vi "PDash - Rename DQMH Module.vi"(9 "New Module Library":path, 10 "Module Info (old)":T1, 11 "Project":refnum<vi>) -> (0 "error out":errorcluster)   [LabVIEW 2019]
doc: "_____\nCreated using DQMH Event Scripter 7.1.0.1447."
uses:
  PantherDashboard Scripting Hooks/Panther Dasboard Scripting Hooks.lvlib
  <vilib>/Delacor/Delacor QMH/Libraries/_Scripting Support/Module Type--enum.ctl
  <vilib>/Delacor/Delacor QMH/Libraries/_Scripting Support/dqmh_lib_DQMH Scripting Support.lvlib
  <vilib>/Delacor/Delacor QMH/Libraries/_Scripting Support/Module Info--cluster.ctl
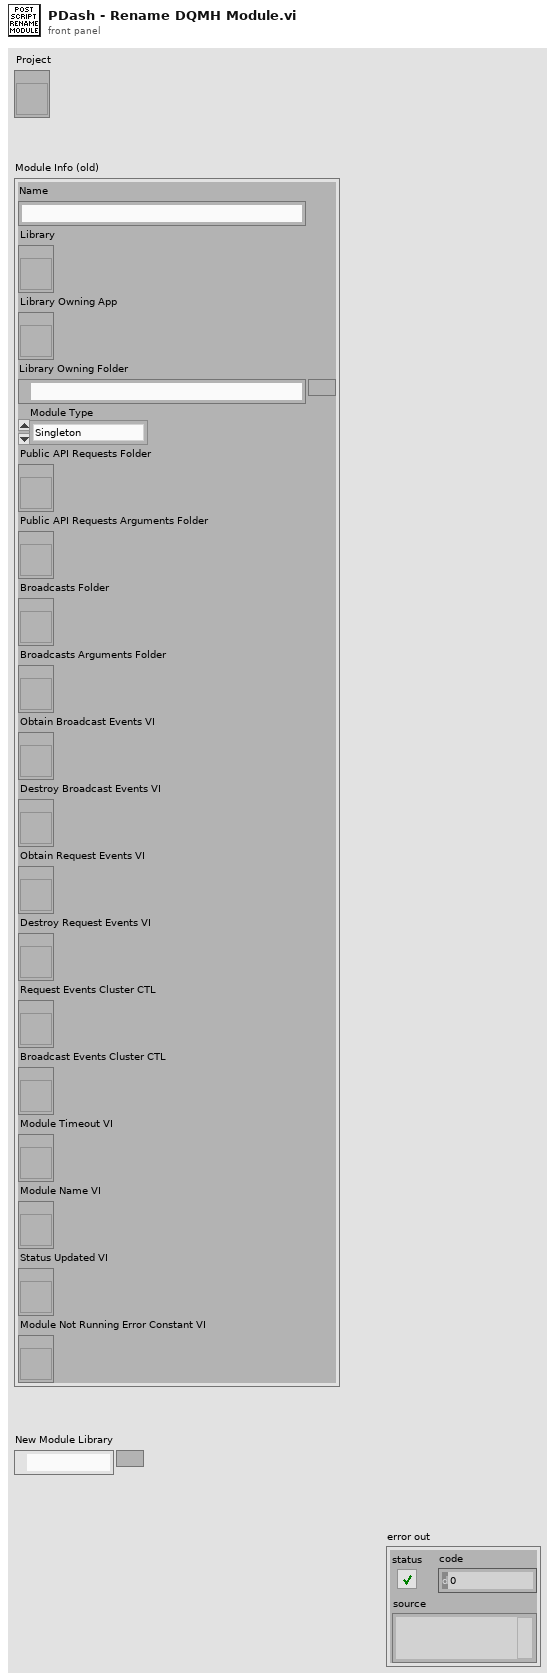
[diagram p1: front panel]
types:
  T1 = typedef "dqmh_lib_DQMH Scripting Support.lvlib/Module Info--cluster.ctl" = cluster{"Name":string, "Library":refnum<vi>, "Library Owning App":refnum<vi>, "Library Owning Folder":path, "Module Type":T2, "Public API Requests Folder":refnum<vi>, "Public API Requests Arguments Folder":refnum<vi>, "Broadcasts Folder":refnum<vi>, "Broadcasts Arguments Folder":refnum<vi>, "Obtain Broadcast Events VI":refnum<vi>, "Destroy Broadcast Events VI":refnum<vi>, "Obtain Request Events VI":refnum<vi>, "Destroy Request Events VI":refnum<vi>, "Request Events Cluster CTL":refnum<vi>, "Broadcast Events Cluster CTL":refnum<vi>, "Module Timeout VI":refnum<vi>, "Module Name VI":refnum<vi>, "Status Updated VI":refnum<vi>, "Module Not Running Error Constant VI":refnum<vi>}
  T2 = typedef "dqmh_lib_DQMH Scripting Support.lvlib/Module Type--enum.ctl" = enum16{"Singleton", "Cloneable"}
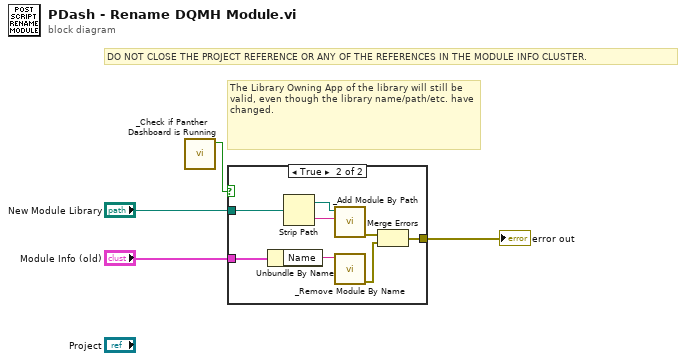
[diagram p0: block diagram]
diagram:
  # "The Library Owning App of the library will still be valid, even though the library name/path/etc. have changed."
  # "DO NOT CLOSE THE PROJECT REFERENCE OR ANY OF THE REFERENCES IN THE MODULE INFO CLUSTER."
  n1 = call "_Check if Panther Dashboard is Running.vi"() -> ("Panther Dashboard is Running?"=w1:bool)  [unwired: 10 in, 1 out]
  n2 = case shown="True" w1 {
    tunnel: "Module Info (old)" -> [_ w9]
    tunnel: "New Module Library" -> [_ w8]
    tunnel: [_ w12] -> w4
    frame False {
    }
    frame True {
      n3 = Unbundle By Name(w9) -> ("Name"=w5:string)
      n4 = Strip Path(path=w8) -> (stripped path=w7:path, name=w6:string)
      n5 = call "_Add Module By Path.vi"("New Module Name"=w6, "New Module Folder"=w7) -> ("error out"=w11:errorcluster)  [unwired: 9 in]
      n6 = call "_Remove Module By Name.vi"("Module Name"=w5) -> ("error out"=w10:errorcluster)  [unwired: 10 in]
      n7 = Merge Errors(w11, w10) -> (w12:errorcluster)
    }
  }
  "error out" <- w4
